vi "RememberBlobLocation.vi"(11 "Target Data":T1) -> (3 "Target Data":T1)   [LabVIEW 2016]
uses:
  Robot Global Data.vi
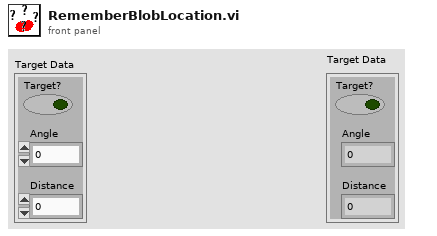
[diagram p1: front panel]
types:
  T1 = cluster{"Target?":bool, "Angle":dbl, "Distance":dbl}
  T2 = cluster{"theta":dbl, "distance":dbl, "x":dbl, "y":dbl}[]
  T3 = cluster{"theta":dbl, "distance":dbl, "x":dbl, "y":dbl}
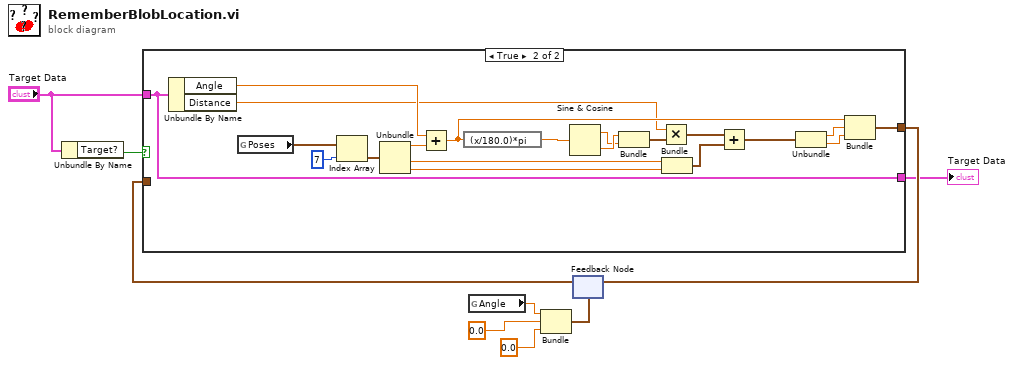
[diagram p0: block diagram]
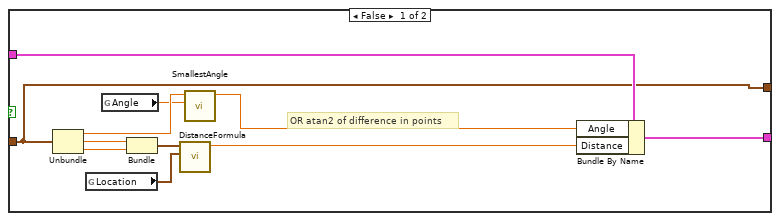
[diagram p2: hidden frame]
diagram:
  n1 = Unbundle By Name("Target Data") -> ("Target?"=w9:bool)
  n2 = global read "Robot Global Data.vi" "Angle"() -> (w6:dbl)
  n3 = Bundle("Angle"=w6, 0.0, 0.0) -> (w5:cluster{"Angle":dbl, dbl, dbl})  [unwired: 1 in]
  n4 = feedback #1(w5) -> (w8:cluster{"Angle":dbl, dbl, dbl})
  n5 = case shown="True" w9 {
    tunnel: "Target Data" -> [w19 w38]
    tunnel: [w16 w21] -> w7
    tunnel: w8 -> [w16 _]
    tunnel: [w18 w38] -> w2
    frame False {
      # "OR atan2 of difference in points"
      n6 = Unbundle(w16) -> ("Angle"=w17:dbl, w14:dbl, w13:dbl)
      n7 = global read "Robot Global Data.vi" "Location"() -> (w11:cluster{"x":dbl, "y":dbl})
      n8 = global read "Robot Global Data.vi" "Angle"() -> (w15:dbl)
      n9 = Bundle(w14, w13) -> (w12:cluster{dbl, dbl})  [unwired: 1 in]
      n10 = call "DistanceFormula.vi"("Point 2"=w11, "Point 1"=w12) -> ("Distance"=w10:dbl)  [unwired: 9 in]
      n11 = call "SmallestAngle.vi"("Angle 2"=w15, "Angle 1"=w17) -> ("Smallest Difference"=w20:dbl)  [unwired: 9 in]
      n12 = Bundle By Name(cluster=w19, "Angle"=w20, "Distance"=w10) -> (w18:T1)
    }
    frame True {
      n13 = Unbundle By Name(w38) -> ("Angle"=w36:dbl, "Distance"=w29:dbl)
      n14 = global read "Robot Global Data.vi" "Poses"() -> (w40:T2)
      n15 = Index Array(array=w40, index=7) -> (element=w37:T3)
      n16 = Unbundle(w37) -> ("theta"=w35:dbl, "x"=w27:dbl, "y"=w26:dbl)  [unwired: 1 out]
      n17 = Add(x=w36, y=w35) -> (x+y=w34:dbl)
      n18 = expression code="(x/180.0)*pi" ("degrees to radians")(w34) -> (w33:dbl)
      n19 = Sine & Cosine(0:w33) -> (1:w31:dbl, 2:w32:dbl)
      n20 = Bundle(w32, w31) -> (w30:cluster{dbl, dbl})  [unwired: 1 in]
      n21 = Multiply(x=w29, y=w30) -> (x*y=w28:cluster{dbl, dbl})
      n22 = Bundle("x"=w27, "y"=w26) -> (w25:cluster{"x":dbl, "y":dbl})  [unwired: 1 in]
      n23 = Add(x=w28, y=w25) -> (x+y=w22:cluster{dbl, dbl})
      n24 = Unbundle(w22) -> (w24:dbl, w23:dbl)
      n25 = Bundle(w34, w24, w23) -> (w21:cluster{dbl, dbl, dbl})  [unwired: 1 in]
    }
  }
  "Target Data" <- w2
  n26 = feedback-in #1(w7) -> ()
